vi "01 - Simple UI.vi"() -> ()   [LabVIEW 2025]
uses:
  <vilib>/measure/NI_MABase.lvlib
  <vilib>/measure/NI_MAPro.lvlib
  <vilib>/measure/maspectr.llb/FFT Spectrum (Mag-Phase) for 1 Chan.vi
  <vilib>/measure/macond.llb/FIR Filter for 1 Chan.vi
  <vilib>/Analysis/4window.llb/windowTd.ctl
  <vilib>/Analysis/NI_AALPro.lvlib
panel:
  out "Waveform Graph 2":waveform(dbl)[](graph)=[{"t0"=timestamp(0 s since 1904-01-01), "dt"=0.001, "Y"=array[1000 elements]}, {"t0"=timestamp(0 s since 1904-01-01), "dt"=0.001, "Y"=array[1000 elements]}]
  in  "optional FIR filter specifications":T1={"PB Gain"=-0.1, "SB Gain"=-60.0, "Scale"=TRUE, "Window"=enum."None"} {"SB Gain" format="%.2p"; "PB Gain" format="%.2p"}
  in  "window":T2=1 items=["Rectangle"=0, "Hanning"=1, "Hamming"=2, "Blackman-Harris"=3, "Exact Blackman"=4, "Blackman"=5, "Flat Top"=6, "4 Term B-Harris "=7, "7 Term B-Harris"=8, "Low Sidelobe"=9, "Blackman Nuttall"=11, "Triangle"=30, "Bartlett-Hanning"=31, "Bohman"=32, "Parzen"=33, "Welch"=34, "Kaiser"=60, "Dolph-Chebyshev"=61, "Gaussian"=62]
  out "Waveform Graph":cluster{"f0":dbl, "df":dbl, "magnitude":dbl[]}[](graph)=[{"f0"=0.0, "df"=1.0, "magnitude"=[6.345230100262783e-05, 8.97481633270632e-05, 8.978813893392327e-05, 8.985741254991784e-05, 8.995989395723975e-05, 9.010093314291706e-05, 9.028719574829896e-05, 9.05265023147129e-05, 9.082763183619701e-05, 9.120009123749832e-05, 9.165385394505914e-05, 9.219907264175114e-05, 9.284577343768569e-05, 9.360354081283999e-05, 9.448120449875894e-05, 9.548654065031289e-05, 9.662599993556468e-05, 9.790447436977789e-05, 9.932511280522798e-05, 0.00010088919212138582, 0.00010259604764225814, 0.00010444306256096748, 0.00010642571262028289, 0.00010853765936571506, 0.00011077088322950808, 0.00011311584662216268, 0.00011556167707229074, 0.00011809636110499217, 0.00012070694076093293, 0.00012337970619065886, 0.00012610037939294195, 0.00012885428572673635, 0.00013162651120270062, 0.00013440204468662676, 0.00013716590500840892, 0.0001399032535815693, 0.00014259949352918183, 0.00014524035652771974, 0.00014781197866068526, 0.00015030096655813382, 0.00015269445501947117, 0.00015498015720090812, 0.00015714640831459412, 0.0001591822036501222, 0.00016107723159302604, 0.00016282190219640925, 0.0001644073717508283, 0.00016582556370503792, 0.0001670691862109057, 0.0001681317465014686, 0.00016900756225879068, 0.0001696917700870244, 0.00017018033117615556, 0.00017047003421792858, 0.00017055849562197184, 0.0001704441570684511, 0.00017012628042973352, 0.000169604940094589, 0.5001688761638524, 0.9998334708191067, 0.5001608602936197, 0.00016551422398564453, 0.0001640042623770181, 0.00016230759904248526, 0.00016042957172068432, 0.00015837618134555926, 0.000156154063454587, 0.00015377045771882805, 0.00015123317572213188, 0.00014855056711984767, 0.00014573148431780373, 0.00014278524581583363, 0.00013972159836138278, 0.00013655067806005782, 0.00013328297058518663, 0.0001299292706222865, 0.0001265006406699011, 0.00012300836930276925, 0.00011946392897686552, 0.00011587893342176221, 0.000112265094627067, 0.0001086341793697326, 0.00010499796516838824, 0.00010136819546601425, 9.775653374764166e-05, 9.417451618852611e-05, 9.063350230258658e-05, 8.714462292724966e-05, 8.37187247408097e-05, 8.036631038558699e-05, 7.709747317062673e-05, 7.392182529304831e-05, 7.084841857794728e-05, 6.788565694254686e-05, 6.504120020537744e-05, 6.232185952708743e-05, 5.9733485749940656e-05, 5.728085319989753e-05, 5.4967543100818696e-05, 5.2795832503851485e-05, 5.0766596349755786e-05, 4.887923164712205e-05, 4.713161339894974e-05, 4.5520091478149374e-05, 4.4039535885908005e-05, 4.268343469039504e-05, 4.1444044689364105e-05, 4.031259002529771e-05, 3.927949935132056e-05, 3.833466848612471e-05, 3.746773340522794e-05, 3.666833818423645e-05, 3.592638403140327e-05, 3.523224840948694e-05, 3.457696684709626e-05, 3.395237375833237e-05, 3.3351201922428085e-05, 3.276714290349378e-05, 3.2194872480726315e-05, 3.1630046152792546e-05, 3.106927009565212e-05, 3.0510052775282382e-05, 2.995074191725757e-05, 2.939045087028165e-05, 2.8828977687472365e-05, 2.8266719568343878e-05, 2.770458471109686e-05, 2.7143903140594314e-05, 2.6586337716761527e-05, 2.603379629112835e-05, 2.548834585189569e-05, 2.4952129474417364e-05, 2.442728694736331e-05, 2.3915880059849394e-05, 2.341982367433751e-05, 2.2940823847087234e-05, 2.248032435186569e-05, 2.2039462976872382e-05, 2.1619038869697653e-05, 2.1219491976024597e-05, 2.084089525287531e-05, 2.0482959849800913e-05, 2.014505288029202e-05, 1.9826226799819515e-05, 1.9525258836711887e-05, 1.924069844053621e-05, 1.897092037959976e-05, 1.8714180958906948e-05, 1.846867485117576e-05, 1.823259022216365e-05, 1.8004160147276495e-05, 1.7781708719548808e-05, 1.7563690686356542e-05, 1.734872388554714e-05, 1.7135614144549893e-05, 1.6923372638021365e-05, 1.6711225962474683e-05, 1.649861937690488e-05, 1.6285213786103116e-05, 1.6070877119895165e-05, 1.585567079435312e-05, 1.5639831956116232e-05, 1.5423752198584193e-05, 1.5207953436632395e-05, 1.4993061613795405e-05, 1.4779778916370417e-05, 1.456885517491445e-05, 1.4361059146469415e-05, 1.4157150384534703e-05, 1.3957852415504797e-05, 1.376382793881165e-05, 1.3575656747606083e-05, 1.3393817018786571e-05, 1.3218670539712342e-05, 1.3050452321998838e-05, 1.2889264901584429e-05, 1.2735077444016805e-05, 1.2587729577427828e-05, 1.244693967431154e-05, 1.2312317113321538e-05, 1.2183377889913565e-05, 1.2059562820303643e-05, 1.1940257506369686e-05, 1.1824813202884584e-05, 1.1712567750925325e-05, 1.1602865803605054e-05, 1.1495077668838547e-05, 1.1388616209273598e-05, 1.1282951368768326e-05, 1.1177622022497513e-05, 1.107224496851339e-05, 1.0966520988053922e-05, 1.0860237994317217e-05, 1.0753271366782932e-05, 1.0645581630455484e-05, 1.0537209689367885e-05, 1.0428269859876554e-05, 1.0318940984104999e-05, 1.0209455925366488e-05, 1.0100089773074706e-05, 9.991147101743065e-06, 9.882948647707861e-06, 9.775817780432056e-06, 9.670067155849916e-06, 9.565985940936914e-06, 9.463827993549313e-06, 9.363801362003758e-06, 9.266059436884397e-06, 9.170694040871132e-06, 9.077730678907426e-06, 8.987126096161589e-06, 8.898768206056336e-06, 8.812478357926668e-06, 8.728015824771828e-06, 8.64508430396091e-06, 8.563340149773158e-06, 8.482401998270802e-06, 8.401861402504132e-06, 8.321294076191487e-06, 8.240271341783112e-06, 8.15837139427033e-06, 8.075190022822448e-06, 7.99035047324918e-06, 7.903512183547313e-06, 7.814378176593926e-06, 7.722700949436064e-06, 7.628286750482231e-06, 7.530998186485147e-06, 7.430755150302552e-06, 7.327534101247661e-06, 7.221365774694276e-06, 7.112331431775526e-06, 7.000557797619155e-06, 6.886210868046268e-06, 6.769488795253867e-06, 6.650614089432109e-06, 6.529825396552302e-06, 6.407369129988938e-06, 6.283491243896256e-06, 6.158429439527905e-06, 6.032406086076499e-06, 5.905622120063759e-06, 5.778252152771561e-06, 5.650440974093389e-06, 5.52230158344327e-06, 5.393914813923969e-06, 5.26533054735773e-06, 5.136570442678807e-06, 5.007632032252344e-06, 4.878493975885125e-06, 4.74912221294082e-06, 4.619476712856877e-06, 4.489518505928467e-06, 4.359216671603439e-06, 4.228554974385448e-06, 4.097537865844927e-06, 3.966195609897416e-06, 3.834588337422202e-06, 3.7028088880893133e-06, 3.5709843540490707e-06, 3.4392762904435497e-06, 3.3078796127279938e-06, 3.177020238913403e-06, 3.0469515809709953e-06, 2.9179500161051776e-06, 2.790309497567718e-06, 2.6643354838295342e-06, 2.5403383791488674e-06, 2.4186266890503868e-06, 2.299500100337164e-06, 2.1832426972893336e-06, 2.070116526124268e-06, 1.9603557146474965e-06, 1.8541613465553476e-06, 1.7516972758118553e-06, 1.6530870465047384e-06, 1.5584120540707722e-06, 1.4677110463706362e-06, 1.3809810122622555e-06, 1.2981794483157727e-06, 1.2192279253362317e-06, 1.1440168087837144e-06, 1.0724109169526464e-06, 1.004255844220614e-06, 9.393846337291096e-07, 8.776244641864925e-07, 8.188030210902548e-07, 7.627542537819571e-07, 7.093232722707855e-07, 6.583702085480101e-07, 6.097729428720004e-07, 5.63428675017393e-07, 5.192543899593976e-07, 4.77186325665591e-07, 4.3717859432850514e-07, 3.992011320104744e-07, 3.63237164726019e-07, 3.2928037230497667e-07, 2.973319186407854e-07, 2.6739749114241094e-07, 2.3948446019739854e-07, 2.1359923012143387e-07, 1.8974480423549585e-07, 1.679185265942686e-07, 1.4810989326402068e-07, 1.302982389140552e-07, 1.1445002953378851e-07, 1.0051545697575368e-07, 8.842413819147563e-08, 7.808009637828176e-08, 6.935694796367838e-08, 6.209520240730569e-08, 5.610420026989693e-08, 5.117056450948054e-08, 4.707275084708437e-08, 4.359843815210609e-08, 4.056010364746054e-08, 3.780518069379545e-08, 3.521971867445888e-08, 3.2726680924641676e-08, 3.0280970390418835e-08, 2.786314266021192e-08, 2.5473150912372156e-08, 2.312484618173337e-08, 2.084151306143243e-08, 1.8652454134235432e-08, 1.659048475345975e-08, 1.4690078649099466e-08, 1.29857398770919e-08, 1.150993012068937e-08, 1.028965586563893e-08, 9.341061898875875e-09, 8.662828948968572e-09, 8.231691957907172e-09, 8.004309335837492e-09, 7.92615114272462e-09, 7.942843683156424e-09, 8.008517244193094e-09, 8.089196550927105e-09, 8.162459850492415e-09, 8.215355785102042e-09, 8.241947720813074e-09, 8.241113824395153e-09, 8.21478557765934e-09, 8.166615711329148e-09, 8.101009732369732e-09, 8.022451453008403e-09, 7.935060992676063e-09, 7.842338573117542e-09, 7.747051076832373e-09, 7.651226324486397e-09, 7.556221142476879e-09, 7.462833426673541e-09, 7.3714335233183335e-09, 7.282093475912047e-09, 7.194702229806626e-09, 7.109056900263204e-09, 7.024929292718286e-09, 6.942107814301215e-09, 6.860419202050505e-09, 6.779735893957865e-09, 6.6999717239621e-09, 6.621074447476481e-09, 6.543015095169077e-09, 6.465778438105272e-09, 6.389355583017103e-09, 6.313738884247097e-09, 6.238919414895732e-09, 6.164885886859541e-09, 6.091625189992738e-09, 6.019123064343491e-09, 5.947365196867062e-09, 5.876337761230497e-09, 5.806028023367579e-09, 5.736424116229623e-09, 5.6675150911261114e-09, 5.599290260373858e-09, 5.531739290921842e-09, 5.464851574031649e-09, 5.398616333341905e-09, 5.333022672424396e-09, 5.26805950362295e-09, 5.203715969448159e-09, 5.139981387416318e-09, 5.076845401522699e-09, 5.0142981876617e-09, 4.952330127015343e-09, 4.890932066733847e-09, 4.830094895462263e-09, 4.769809735239784e-09, 4.710067611696265e-09, 4.6508596350200615e-09, 4.5921768845107535e-09, 4.534010461039222e-09, 4.476351585729636e-09, 4.419191674451713e-09, 4.36252237570273e-09, 4.30633553268274e-09, 4.25062326783064e-09, 4.195377945035818e-09, 4.140591995697055e-09, 4.08625806053249e-09, 4.032368750100488e-09, 3.978916673116383e-09, 3.925894475033722e-09, 3.873294825836123e-09, 3.821110314948969e-09, 3.769333857334239e-09, 3.7179582554081347e-09, 3.6669766683689917e-09, 3.6163824124759055e-09, 3.566168929254583e-09, 3.516329943395994e-09, 3.46685931039834e-09, 3.4177509024460384e-09, 3.368998744922188e-09, 3.3205967914798342e-09, 3.2725390346585195e-09, 3.224819416943163e-09, 3.1774318737292467e-09, 3.13037037698407e-09, 3.0836290107375953e-09, 3.0372018715102197e-09, 2.9910832464714946e-09, 2.9452676123233907e-09, 2.899749564824349e-09, 2.8545239195750015e-09, 2.809585497587635e-09, 2.764929309443744e-09, 2.7205503660685684e-09, 2.6764437492244738e-09, 2.6326044278806006e-09, 2.5890274432802818e-09, 2.5457077627703443e-09, 2.502640391500202e-09, 2.4598203847239374e-09, 2.417242743367249e-09, 2.3749027512175993e-09, 2.3327956800805106e-09, 2.290916884729933e-09, 2.2492620796539886e-09, 2.207826816846575e-09, 2.166606888093835e-09, 2.125598095910662e-09, 2.0847962735472423e-09, 2.0441972625145685e-09, 2.0037969051044392e-09, 1.963590988210712e-09, 1.9235753465070146e-09, 1.883745798371129e-09, 1.8440981951795106e-09, 1.804628501892053e-09, 1.7653327289096017e-09, 1.7262069767147759e-09, 1.6872475204060184e-09, 1.6484507078365441e-09, 1.6098129408814671e-09, 1.5713307900074446e-09, 1.5330007058268569e-09, 1.4948194869663275e-09, 1.4567834034537835e-09, 1.4188893560091551e-09, 1.3811339236187097e-09, 1.3435136919091733e-09, 1.3060254743449097e-09, 1.2686660566821392e-09, 1.2314324258756502e-09, 1.1943216263309772e-09, 1.157330981581519e-09, 1.1204578963119528e-09, 1.083700019793997e-09, 1.047055177886817e-09, 1.0105213964381024e-09, 9.74096947284972e-10, 9.37780194605454e-10, 9.015699644020618e-10, 8.654652922541822e-10, 8.294655551236002e-10, 7.935708196095031e-10, 7.577816094680642e-10, 7.220994199168829e-10, 6.865267221317513e-10, 6.510673601434419e-10, 6.157268082830993e-10, 5.805127756651298e-10, 5.45435748346499e-10, 5.105099113972659e-10, 4.757545693217687e-10, 4.4119576038944265e-10, 4.0686943839390114e-10, 3.728253167265507e-10, 3.3913412742426973e-10, 3.0589787739902596e-10, 2.7326821027378274e-10, 2.41476746596766e-10, 2.108886166424116e-10, 1.8209759145841143e-10, 1.5608813541821734e-10, 1.3447239960018666e-10, 1.1964651728574625e-10]}, ...(2 in all)]
  in  "FIR filter specifications":T3={"Topology"=enum."Equi-ripple FIR", "Type"=enum."Lowpass", "#Taps"=60, "Lower PB"=160.0, "Upper PB"=0.0, "Lower SB"=360.0, "Upper SB"=0.0} {"Lower SB" format="%0.2p"; "Upper SB" format="%0.2p"; "Lower PB" format="%0.2p"; "Upper PB" format="%0.2p"}
  in  "Horizontal Pointer Slide":i32(slide)=59 scale=0.0..500.0
  # "To experiment with configuration\nClick the above button that looks like this"
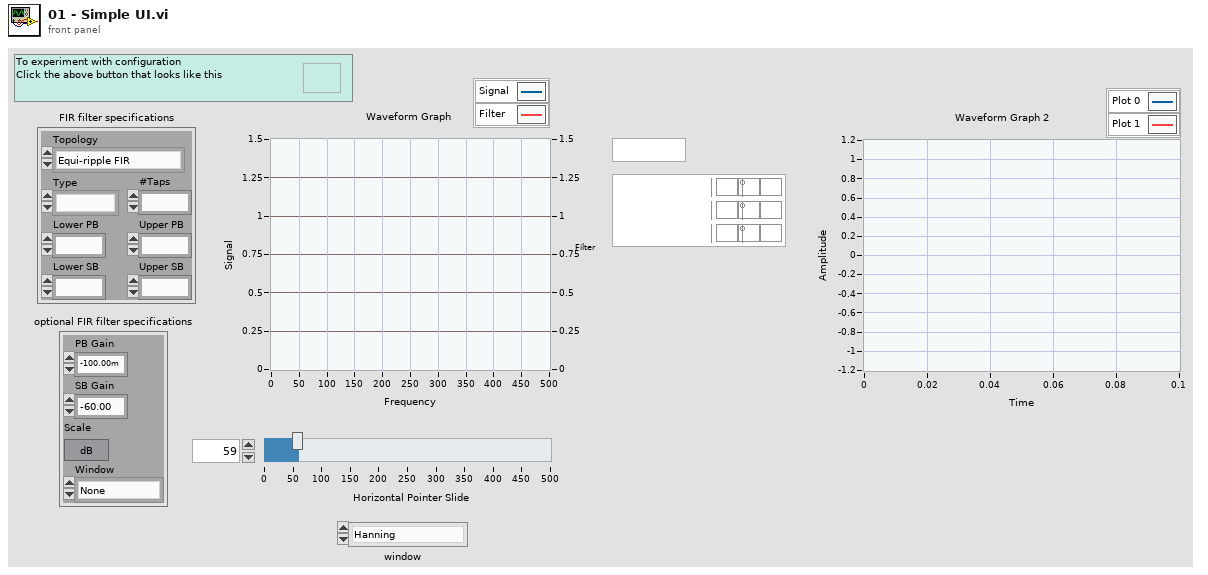
[diagram p1: front panel]
types:
  T1 = cluster{"PB Gain":dbl, "SB Gain":dbl, "Scale":bool, "Window":enum16{"None", "Hanning", "Hamming", "Triangular", "Blackman", "Exact Blackman", "Blackman-Harris", "Kaiser-Bessel", "Flat Top"}}
  T2 = typedef "NI_AALPro.lvlib/windowTd.ctl" = u32
  T3 = cluster{"Topology":enum16{"Off", "FIR by Specification", "Equi-ripple FIR", "Windowed FIR"}, "Type":enum16{"Lowpass", "Highpass", "Bandpass", "Bandstop"}, "#Taps":i32, "Lower PB":dbl, "Upper PB":dbl, "Lower SB":dbl, "Upper SB":dbl}
  T4 = cluster{"magnitude H(w)":cluster{"f0":dbl, "df":dbl, "Mag H(w)":dbl[]}, "phase H(w)":cluster{"f0":dbl, "df":dbl, "Phase H(w)":dbl[]}, "order":i32}
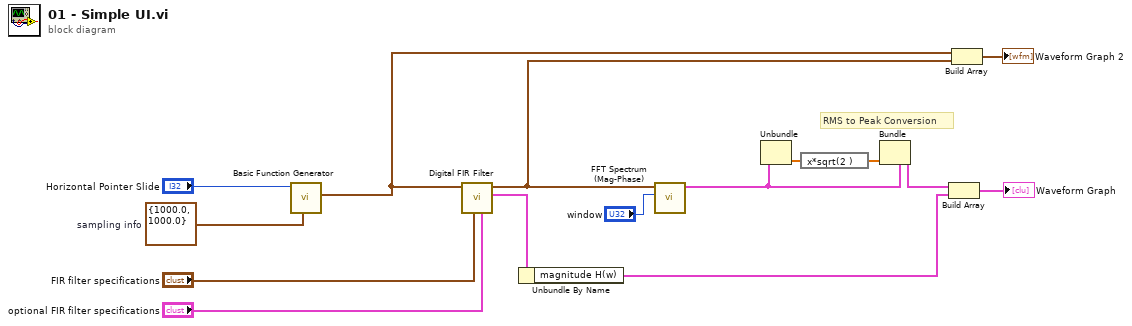
[diagram p0: block diagram]
diagram:
  w11 = cluster{"Fs":dbl, "#s":dbl} {"Fs"=1000.0, "#s"=1000.0}  # sampling info
  # "RMS to Peak Conversion"
  n1 = call <vilib>:"Basic Function Generator.vi"("sampling info"=w11, "frequency"="Horizontal Pointer Slide") -> ("signal out"=w9:waveform(dbl))  [unwired: 7 in, 2 out]
  n2 = call-poly <vilib>:"Digital FIR Filter.vi"("optional FIR filter specifications"="optional FIR filter specifications", "FIR filter specifications"="FIR filter specifications", "signal in"=w9) -> ("filter information"=w13:T4, "signal out"=w7:waveform(dbl))  [unwired: 6 in, 1 out]
  n3 = Unbundle By Name(w13) -> ("magnitude H(w)"=w1:cluster{"f0":dbl, "df":dbl, "Mag H(w)":dbl[]})
  n4 = call-poly <vilib>:"FFT Spectrum (Mag-Phase).vi"("window"="window", "time signal"=w7) -> ("magnitude"=w5:cluster{"f0":dbl, "df":dbl, "magnitude":dbl[]})  [unwired: 5 in, 4 out]
  n5 = Unbundle(w5) -> ("magnitude"=w3:dbl[])  [unwired: 2 out]
  n6 = expression code="x*sqrt(2 )"(w3) -> (w2:dbl[])
  n7 = Bundle(cluster=w5, "magnitude"=w2) -> (w4:cluster{"f0":dbl, "df":dbl, "magnitude":dbl[]})  [unwired: 2 in]
  n8 = Build Array(w4, w1) -> (→"Waveform Graph":cluster{"f0":dbl, "df":dbl, "Mag H(w)":dbl[]}[])
  n9 = Build Array(w9, w7) -> (→"Waveform Graph 2":waveform(dbl)[])
